vi "PicoScope6000aUnitInfo.vi"(7 "Mode":u16(ring) items=["Dialog On Error", "no dialog - CloseUnit and Stop", "no dialog - Continue", "no dialog - Stop"], 8 "error in (no error)":errorcluster, 11 "handle in":i16) -> (0 "error out":errorcluster, 2 "Unit Info":T1, 3 "handle out":i16)   [LabVIEW 2010]
doc: "Returns Driver and Unit Information"
uses:
  ps6000a.dll
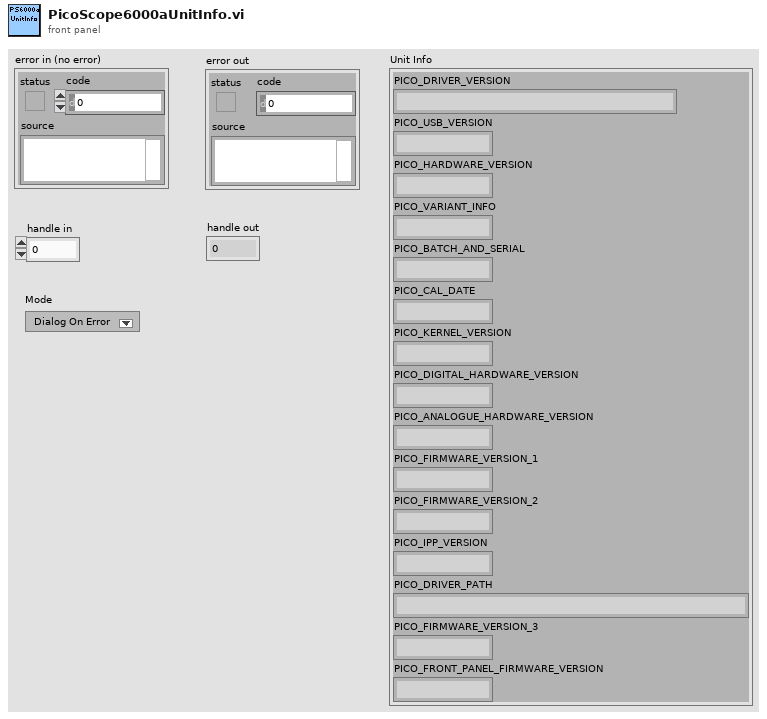
[diagram p1: front panel]
types:
  T1 = cluster{"PICO_DRIVER_VERSION":string, "PICO_USB_VERSION":string, "PICO_HARDWARE_VERSION":string, "PICO_VARIANT_INFO":string, "PICO_BATCH_AND_SERIAL":string, "PICO_CAL_DATE":string, "PICO_KERNEL_VERSION":string, "PICO_DIGITAL_HARDWARE_VERSION":string, "PICO_ANALOGUE_HARDWARE_VERSION":string, "PICO_FIRMWARE_VERSION_1":string, "PICO_FIRMWARE_VERSION_2":string, "PICO_IPP_VERSION":string, "PICO_DRIVER_PATH":string, "PICO_FIRMWARE_VERSION_3":string, "PICO_FRONT_PANEL_FIRMWARE_VERSION":string}
  T2 = cluster{"status":bool, "code":u32, "source":string}
  T3 = cluster{"[0]":string, "[1]":string, "[2]":string, "[3]":string, "[4]":string, "[5]":string, "[6]":string, "[7]":string, "[8]":string, "[9]":string, "[10]":string, "[11]":string, "[12]":string, "[13]":string, "[14]":string}
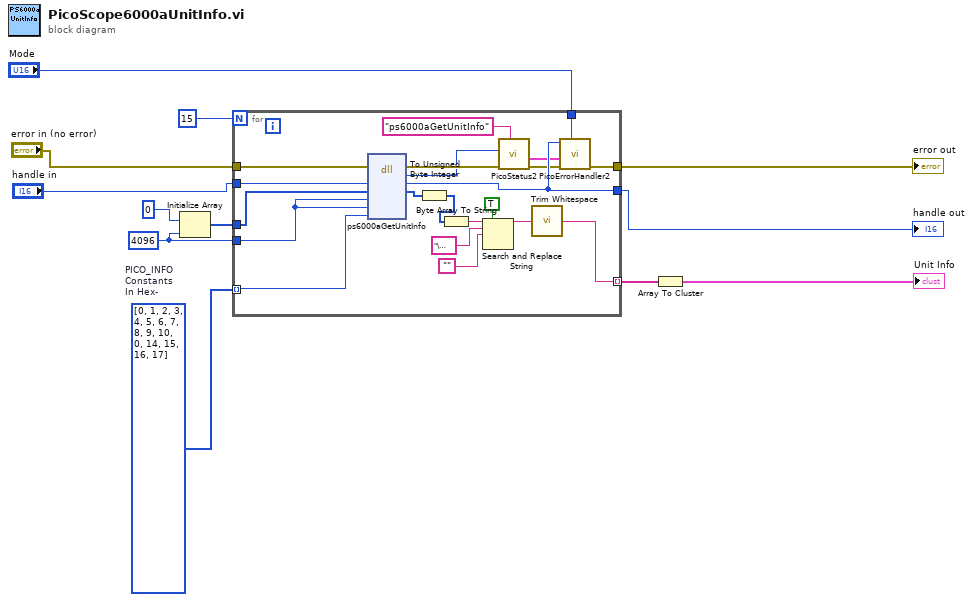
[diagram p0: block diagram]
diagram:
  w4 = i16 4096 ("requiredSize")
  w7 = 15  # PICO_INFO Constants In Hex-
  n1 = Initialize Array(i8 0 ("element"), w4) -> (w6:i8[])
  n2 = for {
    N: w7 -> [_]
    tunnel: "error in (no error)" -> [w27]
    tunnel: [w21] -> w9
    tunnel: w6 -> [w28]
    tunnel: "handle in" -> [w26]
    tunnel: w4 -> [w25]
    tunnel: [w20] -> w10
    tunnel: u32[] [0, 1, 2, 3, 4, 5, 6, 7, 8, 9, 10, 0, 14, 15, 16, 17] ("initialized array") -> [w22] mode=indexing
    tunnel: [w19] -> w3 mode=indexing
    tunnel: "Mode" -> [w13]
    n3 = dll-call lib="ps6000a.dll" fn="ps6000aGetUnitInfo"(error in=w27, "handle"=w26, "string"=w28, "stringLength"=w25, "requiredSize"=w25, "deviceInfo"=w22) -> (error out=w17:errorcluster, "PICO_STATUS"=w14:u32, "handle"=w20:i16, "string"=w24:i8[])  [unwired: 5 in, 1 out]
    n4 = To Unsigned Byte Integer(number=w24) -> (unsigned 8bit integer=w23:u8[])
    n5 = Byte Array To String(unsigned byte array=w23) -> (string=w32:string)
    n6 = Search and Replace String(replace all?=TRUE ("replace all? (F)"), input string=w32, search string="\u0000", replace string="") -> (result string=w31:string)  [unwired: 4 in, 3 out]
    n7 = call "PicoStatus2.vi"("PICO source"="ps6000aGetUnitInfo" ("source"), "Error in"=w17, "PICO STATUS"=w14) -> ("error out"=w18:errorcluster, "PICO_STATUS out"=w16:T2)  [unwired: 5 in]
    n8 = call <vilib>:"Trim Whitespace.vi"("string"=w31) -> ("trimmed string"=w19:string)  [unwired: 1 in]
    n9 = call "PicoErrorHandler2.vi"("Mode"=w13, "error in (no error)"=w18, "PICO_STATUS in"=w16, "handle In"=w20) -> ("error out"=w21:errorcluster)  [unwired: 7 in]
  }
  "error out" <- w9
  "handle out" <- w10
  n10 = Array To Cluster(array=w3) -> (cluster=→"Unit Info":T3)
